vi "input variable.vi"() -> ()   [LabVIEW 2016, in "超标留样集成.lvlib" / "DR803M4.lvlib"]
uses:
  DR803M4.lvlib
  <vilib>/Plasmionique/MB Master/MB_Master_Serial/MB_Master_Serial.lvclass
panel:
  out "流程中":bool
  out "超标留样信号":bool
  in  "信息簇":T1 {"采样模式选择" items=["定时留样", "时间等比例", "同步留样", "外控留样", "超标留样"]; "启停" items=["停止", "启动"]; "采样器进程" items=["待机"=1, "采样瓶排空"=2, "采样瓶润洗"=5, "进样"=6, "取样"=8, "取样管排空"=9]; "门禁标志" items=["关闭", "打开"]; "远程留样" items=["停止", "留样"]}
  in  "MB_Serial session":refnum<class "MB_Master_Serial.lvclass">
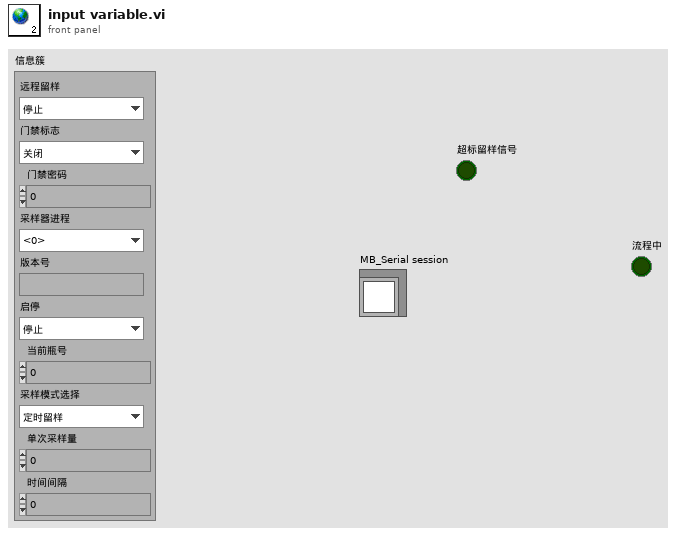
[diagram p1: front panel]
types:
  T1 = cluster{"远程留样":u16, "门禁标志":u16, "门禁密码":u32, "采样器进程":u16, "版本号":string, "启停":u16, "当前瓶号":u16, "采样模式选择":u16, "单次采样量":u16, "时间间隔":u16}
diagram:
